vi "append_to_log.vi"(5 "data_type":T1, 7 "dims":T2, 8 "error in (no error)":errorcluster, 9 "Location":string, 10 "Data":variant, 11 "raw_stream_logger in":refnum<class "raw_stream_logger.lvclass">) -> (0 "error out":errorcluster, 3 "raw_stream_logger out":refnum<class "raw_stream_logger.lvclass">)   [LabVIEW 2015, in "raw_stream_logger.lvclass"]
uses:
  raw_stream_logger.lvclass
  Data Logger Class/data_dimensionality.ctl
  Data Logger Class/logger_data_types.ctl
  raw_stream_logger.lvclass/raw_stream_logger.ctl
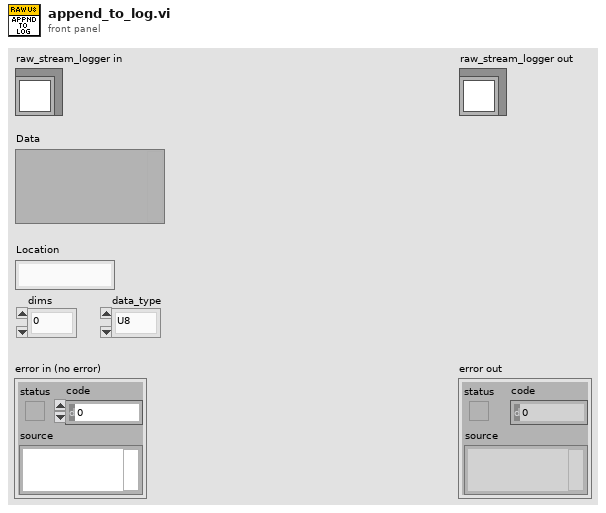
[diagram p1: front panel]
types:
  T1 = typedef "logger_data_types.ctl" = enum16{"U8", "I8", "U16", "I16", "U32", "I32", "DBL", "String"}
  T2 = typedef "data_dimensionality.ctl" = enum16{"0", "1", "2"}
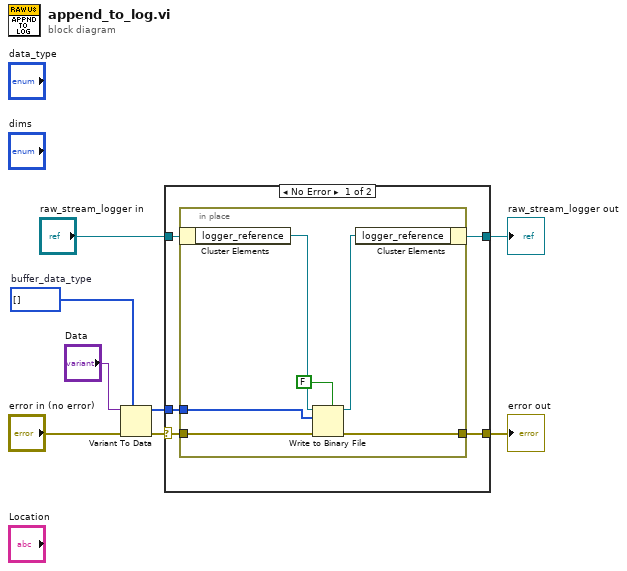
[diagram p0: block diagram]
diagram:
  w6 = u8[] []  # buffer_data_type
  n1 = Variant To Data(error in="error in (no error)", type=w6, Variant="Data") -> (data=w7:u8[], error out=w4:errorcluster)
  n2 = case shown="No Error" w4 {
    selector: w4 -> [w10 w20]
    tunnel: w7 -> [w11 _]
    tunnel: "raw_stream_logger in" -> [w13 w21]
    tunnel: [w12 w21] -> w2
    tunnel: [w9 w20] -> w1
    frame No Error {
      n3 = in-place {
        in-place-border: w11 -> [w17]
        in-place-border: w10 -> [w16]
        in-place-border: [w15] -> w9
        n4 = in-place-cluster #1(w13) -> ("logger_reference"=w19:refnum<file>)
        n5 = Write to Binary File(file (use dialog)=w19, data=w17, error in=w16, 5:FALSE ("prepend array or string size? (T)")) -> (refnum out=w18:refnum<file>, error out=w15:errorcluster)  [unwired: 2 in, 1 out]
        n6 = in-place-cluster #1("logger_reference"=w18) -> (w12:refnum<class "raw_stream_logger.lvclass">)
      }
    }
    frame Error {
    }
  }
  "error out" <- w1
  "raw_stream_logger out" <- w2
